vi "REPORT_PBATCH_prepare_header_for_pdf.vi"(11 "REPORT_PBATCH_all_info":T1) -> (3 "report_header":string[][](array[string]))   [LabVIEW 2019]
uses:
  typedef/REPORT_PBATCH_all_info.ctl
  DATES/typedef/REPORT_DATES_statuses.ctl
  _misc/AULocalize/SubVIs/Get Localized Phrase Compact Interface 1D.vi
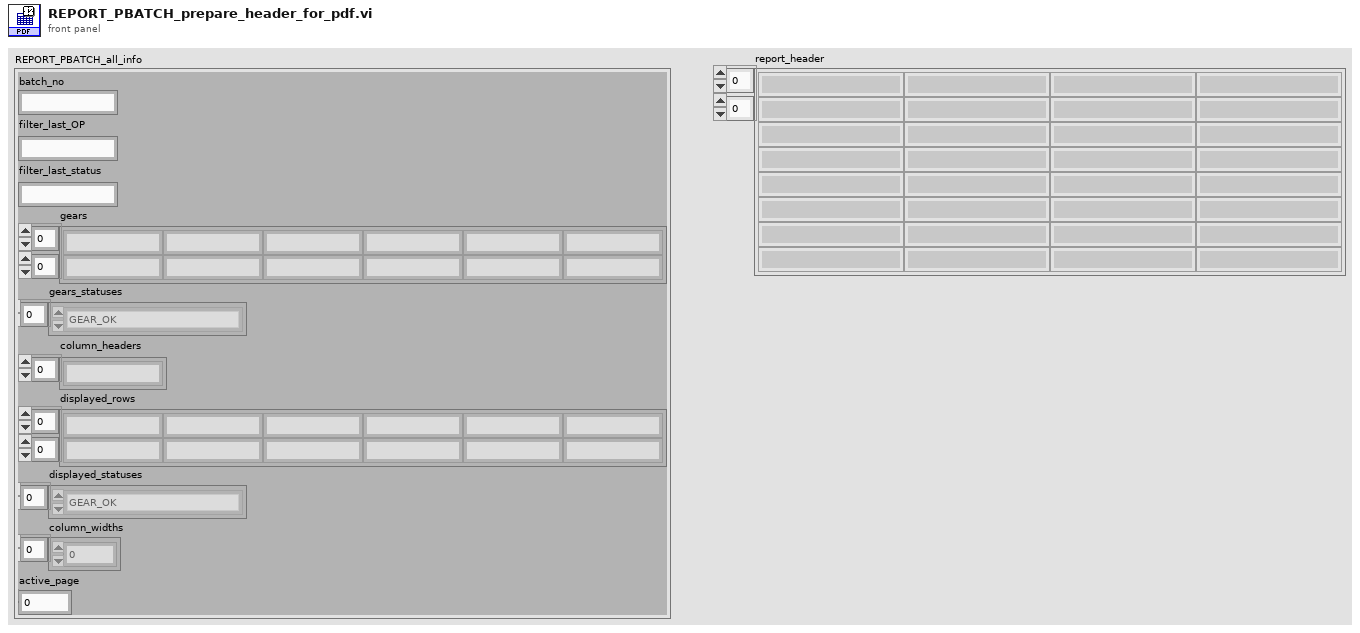
[diagram p1: front panel]
types:
  T1 = typedef "REPORT_PBATCH_all_info.ctl" = cluster{"batch_no":string, "filter_last_OP":string, "filter_last_status":string, "gears":string[][], "gears_statuses":T2[], "column_headers":string[], "displayed_rows":string[][], "displayed_statuses":T2[], "column_widths":i16[], "active_page":i32}
  T2 = typedef "REPORT_DATES_statuses.ctl" = enum16{"GEAR_OK", "GEAR_NOK", "GEAR_interrupted", "GEAR_in_operation", "GEAR_unexpected"}
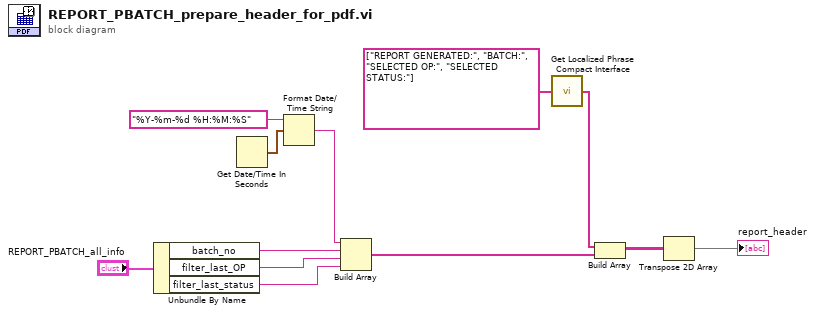
[diagram p0: block diagram]
diagram:
  n1 = Unbundle By Name("REPORT_PBATCH_all_info") -> ("batch_no"=w5:string, "filter_last_OP"=w4:string, "filter_last_status"=w3:string)
  n2 = Get Date/Time In Seconds() -> (seconds since 1Jan1904=w11:timestamp)
  n3 = Format Date/Time String(time format string (%c)="%Y-%m-%d %H:%M:%S", seconds (now)=w11) -> (date/time string=w2:string)  [unwired: 1 in]
  n4 = Build Array(w2, w5, w4, w3) -> (w6:string[])
  n5 = call-poly "Get Localized Phrase Compact Interface.vi"("Key"=string[] ["REPORT GENERATED:", "BATCH:", "SELECTED OP:", "SELECTED STATUS:"]) -> ("Translated Phrase"=w1:string[])
  n6 = Build Array(w1, w6) -> (w9:string[][])
  n7 = Transpose 2D Array(2D array=w9) -> (transposed array=→"report_header":string[][])
